vi "Update CW data.vi"(5 "Sample Array":u32[](array[numeric])) -> (1 "Ref mean":dbl)   [LabVIEW 2020]
uses:
  <vilib>/Analysis/NI_AALBase.lvlib
  <vilib>/Analysis/baseanly.llb/Mean (DBL).vi
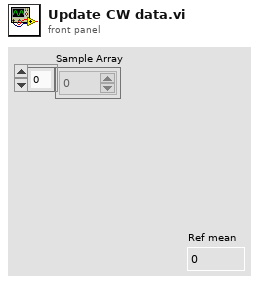
[diagram p1: front panel]
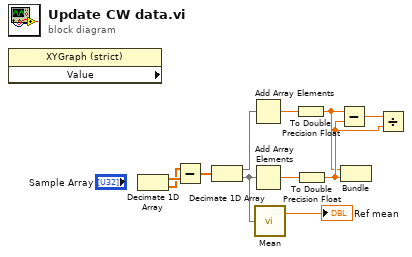
[diagram p0: block diagram]
diagram:
  n1 = property on="Property Node" class="XYGraph (strict)" props=["Value"]() -> ()  [unwired: 2 in, 3 out]
  n2 = Decimate 1D Array() -> (w5:dbl[], w4:dbl[])  [unwired: 1 in]
  n3 = Subtract(x=w4, y=w5) -> (x-y=w6:dbl[])
  n4 = Decimate 1D Array(w6) -> (w7:dbl[], w10:dbl[])
  n5 = Add Array Elements(numeric array=w7) -> (sum=w8:dbl)
  n6 = Add Array Elements(numeric array=w10) -> (sum=w9:dbl)
  n7 = call-poly <vilib>:"Mean.vi"("X"=w10) -> ("mean"=→"Ref mean":dbl)  [unwired: 1 out]
  n8 = To Double Precision Float(number=w8) -> (double precision float=w1:dbl)
  n9 = To Double Precision Float(number=w9) -> (double precision float=w2:dbl)
  n10 = Subtract(x=w1, y=w2) -> (x-y=w11:dbl)
  n11 = Bundle(w1, w2) -> ()  [unwired: 1 in, 1 out]
  n12 = Divide(x=w11, y=w2) -> ()  [unwired: 1 out]
